vi "Load Tests.vi"(8 "error in (no error)":errorcluster, 10 "Tests":string[](array[string]), 11 "Execution UI In":refnum<class "Execution UI.lvclass">) -> (0 "error out":errorcluster, 3 "Execution UI Out":refnum<class "Execution UI.lvclass">)   [LabVIEW 2020, in "Execution UI.lvclass"]
uses:
  Execution UI.lvclass
  Execution UI.lvclass/Execution UI.ctl
  Test Suite/LUnit Test Suite.lvclass
  Test Suite/LUnit Test Suite.lvclass/LUnit Test Suite.ctl
  Test Case/LUnit Test Case.lvclass/LUnit Test Case.ctl
  Test Case/Public/Accessors/Read Enabled Test Methods.vi
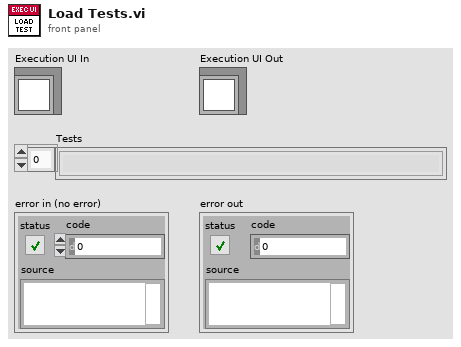
[diagram p1: front panel]
types:
  T1 = typedef "Execution UI.lvclass/Execution State.ctl" = enum16{"Idle", "Running"}
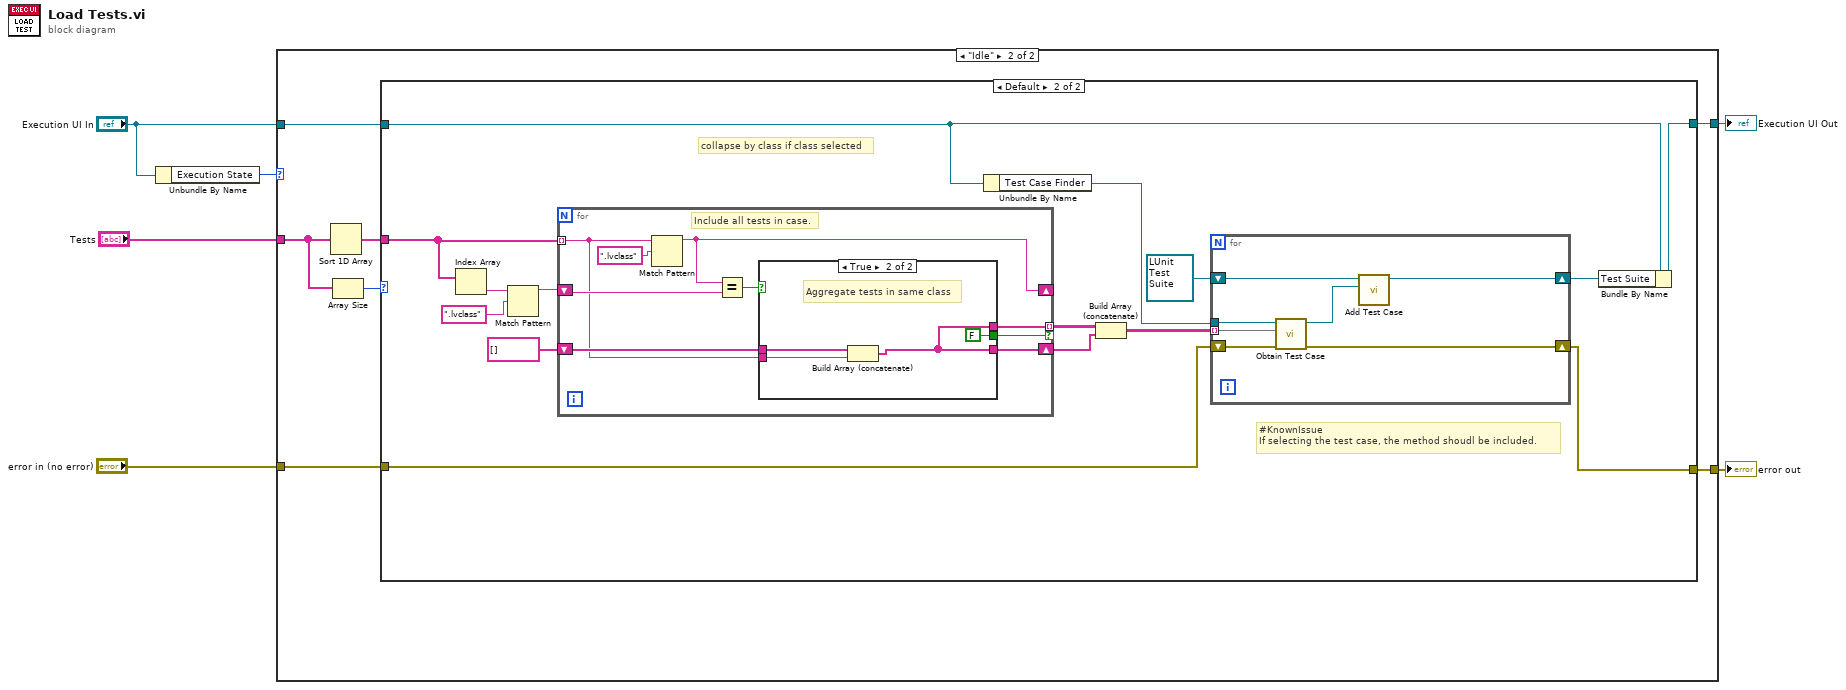
[diagram p0: block diagram]
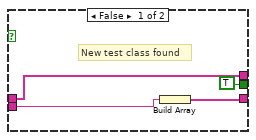
[diagram p4: hidden frame]
diagram:
  n1 = Unbundle By Name("Execution UI In") -> ("Execution State"=w1:T1)
  n2 = case shown="\"Idle\"" w1 {
    tunnel: [w8 w15] -> w6
    tunnel: [w7 w14] -> w5
    tunnel: "error in (no error)" -> [w7 w13]
    tunnel: "Tests" -> [_ w12]
    tunnel: "Execution UI In" -> [w8 w9]
    frame "Running" {
    }
    frame "Idle" {
      n3 = Sort 1D Array(array=w12) -> (sorted array=w10:string[])
      n4 = Array Size(array=w12) -> (size(s)=w11:i32)
      n5 = case shown="Default" w11 {
        tunnel: [w17 w32] -> w15
        tunnel: w9 -> [w17 w19]
        tunnel: [w16 w22] -> w14
        tunnel: w13 -> [w16 w21]
        tunnel: w10 -> [_ w20]
        frame 0 {
        }
        frame Default {
          # "#KnownIssue\nIf selecting the test case, the method shoudl be included."
          # "collapse by class if class selected"
          n6 = Index Array(array=w20) -> (element=w26:string)  [unwired: 1 in]
          n7 = Match Pattern(string=w26, regular expression=".lvclass") -> (before substring=w25:string)  [unwired: 1 in, 3 out]
          n8 = for {
            tunnel: w20 -> [w43] mode=indexing
            shift-right: [w46] -> _
            shift-left: w25 -> [w47]
            shift-right: [w42] -> w28
            shift-left: string[] [] ("String") -> [w44]
            tunnel: [w40] -> w30 mode=indexing if=w41
            # "Include all tests in case."
            n9 = Match Pattern(string=w43, regular expression=".lvclass") -> (before substring=w46:string)  [unwired: 1 in, 3 out]
            n10 = Equal?(x=w46, y=w47) -> (x = y?=w45:bool)
            n11 = case shown="True" w45 {
              tunnel: w43 -> [w51 w56]
              tunnel: w44 -> [w49 w55]
              tunnel: [w52 w53] -> w42
              tunnel: [TRUE FALSE] -> w41
              tunnel: [w49 w53] -> w40
              frame False {
                # "New test class found"
                n12 = Build Array(w51) -> (w52:string[])
              }
              frame True {
                # "Aggregate tests in same class"
                n13 = Build Array (concatenate)(w55, w56) -> (w53:string[])
              }
            }
          }
          n14 = Unbundle By Name(w19) -> ("Test Case Finder"=w18:refnum<class "Test Finder.lvclass">)
          n15 = Build Array (concatenate)(w30, w28) -> (w29:string[][])
          n16 = for {
            tunnel: w29 -> [w34] mode=indexing
            shift-right: [w35] -> w23
            shift-left: refnum<class "LUnit Test Suite.lvclass"> refnum ("Test Suite In") -> [w39]
            shift-right: [w33] -> w22
            shift-left: w21 -> [w37]
            tunnel: w18 -> [w36]
            n17 = call "Obtain Test Case.vi"("error in (no error)"=w37, "Test class and methods"=w34, "Test Finder"=w36) -> ("error out"=w33:errorcluster, "Test Case"=w38:refnum<class "LUnit Test Case.lvclass">)  [unwired: 7 in]
            n18 = call "Add Test Case.vi"("Test Case to add"=w38, "Test Suite In"=w39) -> ("Test Suite Out"=w35:refnum<class "LUnit Test Suite.lvclass">)  [unwired: 9 in]
          }
          n19 = Bundle By Name(cluster=w19, "Test Suite"=w23) -> (w32:refnum<class "Execution UI.lvclass">)
        }
      }
    }
  }
  "error out" <- w5
  "Execution UI Out" <- w6
